vi "MoveForward.vi"() -> ()   [LabVIEW 2019]
uses:
  MotorsGlobal.vi
panel:
  in  "Setpoint":dbl
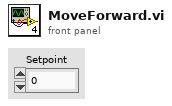
[diagram p1: front panel]
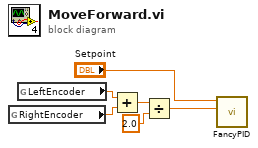
[diagram p0: block diagram]
diagram:
  n1 = global read "MotorsGlobal.vi" "RightEncoder"() -> (w5:dbl)
  n2 = global read "MotorsGlobal.vi" "LeftEncoder"() -> (w6:dbl)
  n3 = Add(x=w6, y=w5) -> (x+y=w4:dbl)
  n4 = Divide(x=w4, y=2.0) -> (x/y=w2:dbl)
  n5 = call "FancyPID.vi"("Process variable"=w2, "Setpoint"="Setpoint") -> ()  [unwired: 9 in, 1 out]
